vi "Analog Mapping Query.vi"(8 "error in (no error)":errorcluster) -> (0 "error out":errorcluster, 2 "AnalogChannels":u8[](array[numeric]))   [LabVIEW 2020, in "FirmataClient.lvlib"]
doc: "VI that will request the analog mapping of pins, i.e. which pins are A0, A1, A2,..."
uses:
  FirmataClient.lvlib
panel:
  in  "Queue Name":string="firmata-serial-communication"
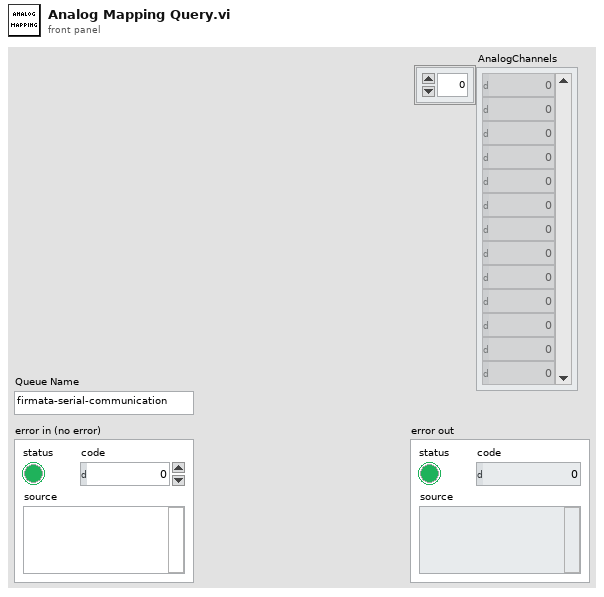
[diagram p1: front panel]
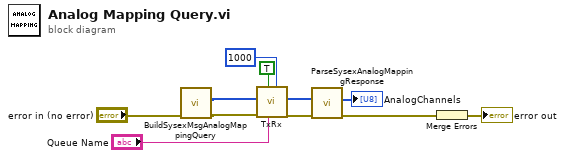
[diagram p0: block diagram]
diagram:
  n1 = call "BuildSysexMsgAnalogMappingQuery.vi"("error in"="error in (no error)") -> ("error out"=w5:errorcluster, "GetAnalogMappingMessage"=w4:u8[])  [unwired: 7 in, 2 out]
  n2 = call "TxRx.vi"("Reply Timeout Ms"=1000, "Queue Name"="Queue Name", "Wait For Reply?"=TRUE, "error in"=w5, "Message"=w4) -> ("error out"=w2:errorcluster, "Reply"=w3:u8[])  [unwired: 5 in]
  n3 = call "ParseSysexAnalogMappingResponse.vi"("error in"=w2, "Sysex Message"=w3) -> ("error out"=w10:errorcluster, "AnalogChannels"=→"AnalogChannels":u8[])  [unwired: 7 in, 1 out]
  n4 = Merge Errors(w10) -> (→"error out":errorcluster)
